vi "NanoDropInterp.vi"() -> ()   [LabVIEW 2022 SP3]
uses:
  <vilib>/gmath/NI_Gmath.lvlib
  <vilib>/Analysis/NI_AALPro.lvlib
  <vilib>/Analysis/NI_AALBase.lvlib
panel:
  in  "Threshol values":dbl[](array[numeric])=[20.0, 30.0]
  in  "delta":dbl
  in  "Cal":string="20\t-0.47978\n40\t-0.89772\n60\t-1.28062\n80\t-1.51509\n100\t-1.73927\n120\t-2.04589\n140\t-2.62307\n160\t-3.32393\n180\t-3.88565\n200\t-4.48344\n220\t-4.98332\n240\t-5.39044\n260\t-5.87486\n280\t-6.95707\n300\t-7.65792\n320\t-8.15265\n340\t-8.31756\n360\t-8.86382\n380\t-8.8329\n400\t-9.08026\n"
  out "Pressure threshold":dbl[][](array[numeric])
  out "Output to cut and paste":string
  out "Interp output":dbl[][](array[numeric])
  in  "shift":dbl
  in  "steps":i32
  in  "Paste tab data":string
  out "Input array":dbl[][](array[numeric])
  # "average and SD are last columns"
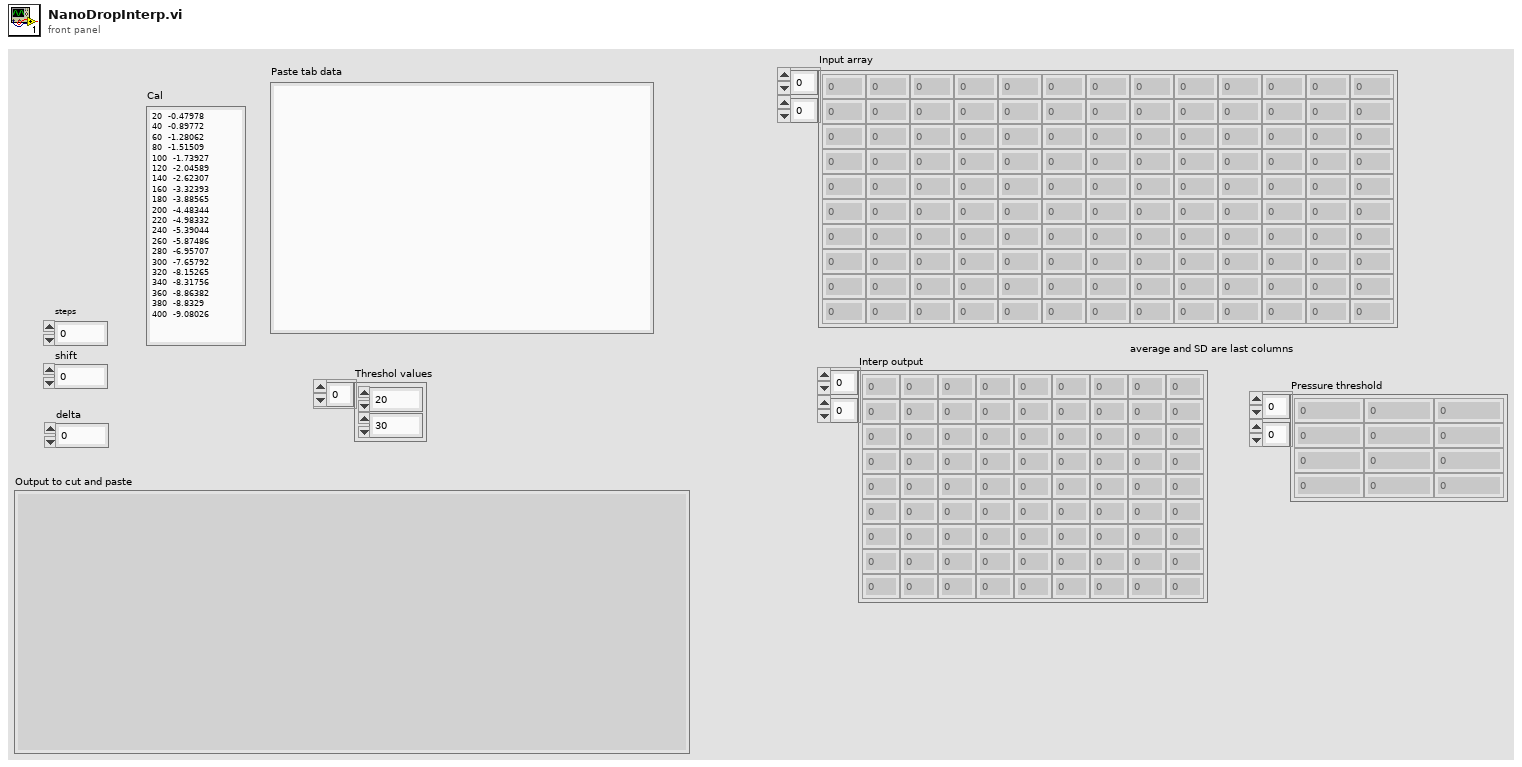
[diagram p1: front panel]
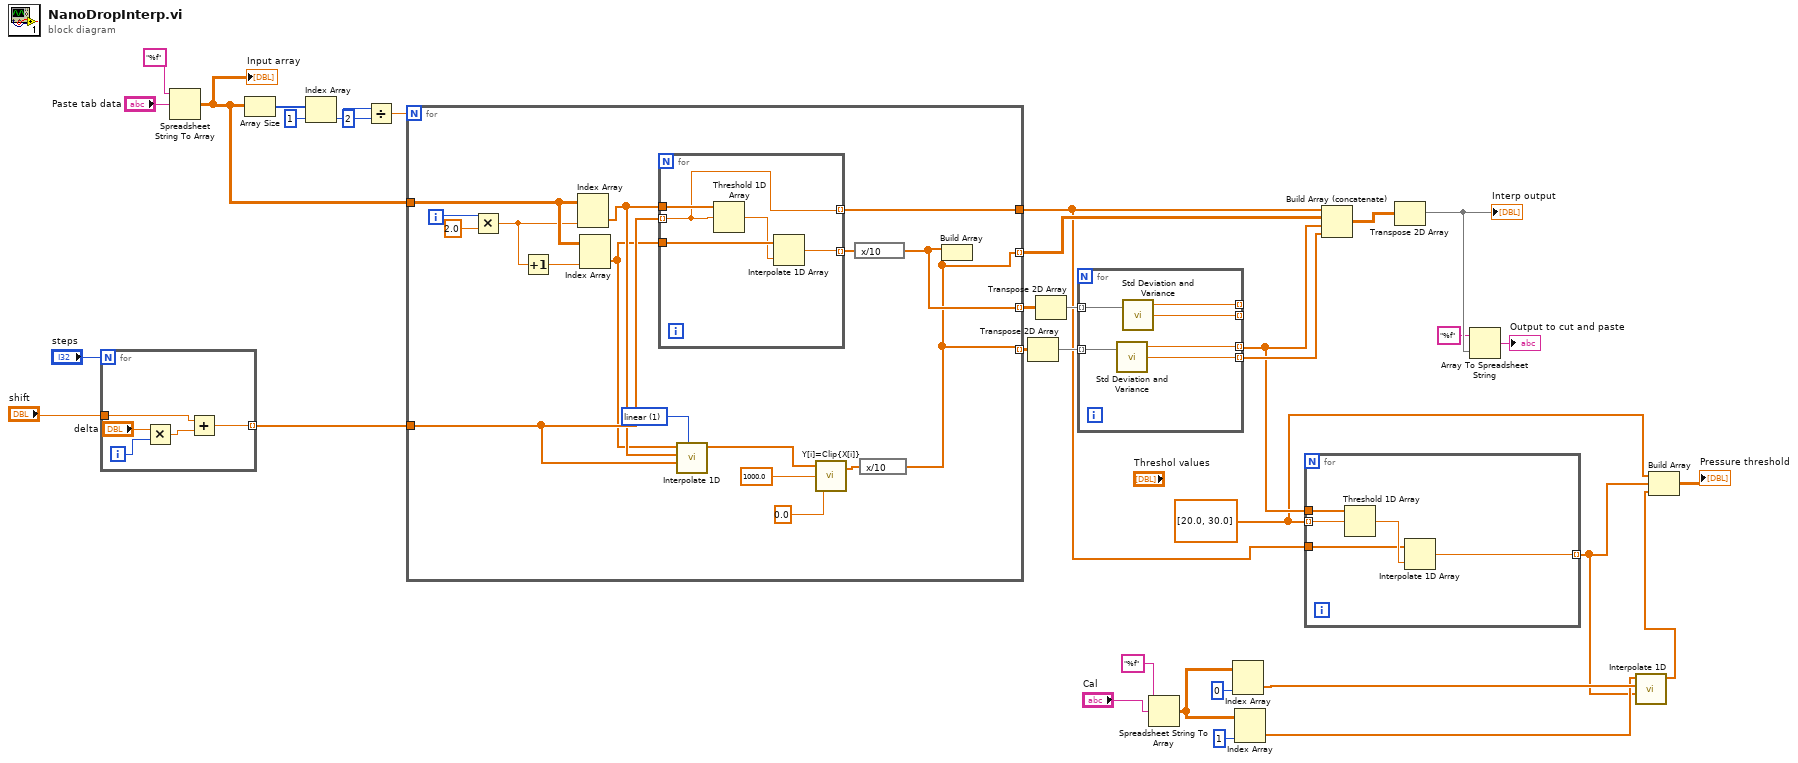
[diagram p0: block diagram]
diagram:
  w11 = dbl[] [20.0, 30.0]
  n1 = for {
    N: "steps" -> [_]
    tunnel: "shift" -> [w37]
    tunnel: [w36] -> w24 mode=indexing
    i -> [w39]
    n2 = Multiply(x="delta", y=w39) -> (x*y=w38:dbl)
    n3 = Add(x=w37, y=w38) -> (x+y=w36:dbl)
  }
  n4 = Spreadsheet String To Array(format string="%f", spreadsheet string="Paste tab data") -> (array=w27:dbl[][])  [unwired: 2 in]
  "Input array" <- w27
  n5 = Array Size(array=w27) -> (size(s)=w32:i32[])
  n6 = Index Array(array=w32, index=1) -> (element=w30:i32)
  n7 = Divide(x=w30, y=2) -> (x/y=w28:dbl)
  n8 = for {
    N: w28 -> [_]
    tunnel: w27 -> [w54]
    tunnel: w24 -> [w51]
    tunnel: [w40] -> w21 mode=indexing
    tunnel: [w40] -> w22 mode=indexing
    tunnel: [w42] -> w23 mode=indexing
    tunnel: [w44] -> w12
    i -> [w55]
    w41 = 1 items=["nearest", "linear", "spline", "cubic Hermite", "Lagrange"] ("method")
    n9 = Multiply(x=w55, y=2.0) -> (x*y=w53:dbl)
    n10 = Increment(x=w53) -> (x+1=w52:dbl)
    n11 = Index Array(array=w54, index (col)=w53) -> (element=w50:dbl[])  [unwired: 1 in]
    n12 = Index Array(array=w54, index (col)=w52) -> (element=w49:dbl[])  [unwired: 1 in]
    n13 = for {
      tunnel: w50 -> [w61]
      tunnel: w51 -> [w58] mode=indexing
      tunnel: w49 -> [w60]
      tunnel: [w59] -> w43 mode=indexing
      tunnel: [w58] -> w44 mode=indexing
      n14 = Threshold 1D Array(2:w58, 3:w61) -> (0:w57:dbl)  [unwired: 1 in]
      n15 = Interpolate 1D Array(1:w57, 2:w60) -> (0:w59:dbl)
    }
    n16 = call <vilib>:"Interpolate 1D.vi"("method"=w41, "xi"=w51, "X"=w50, "Y"=w49) -> ("yi"=w48:dbl[])  [unwired: 5 in, 2 out]
    n17 = call <vilib>:"Y[i]=Clip{X[i]}.vi"("lower limit"=0.0, "upper limit"=1000.0, "Input Array"=w48) -> ("Clipped Array"=w45:dbl[])  [unwired: 1 out]
    n18 = expression code="x/10"(w43) -> (w42:dbl[])
    n19 = expression code="x/10"(w45) -> (w40:dbl[])
    n20 = Build Array(w42, w40) -> ()  [unwired: 1 out]
  }
  n21 = Transpose 2D Array(2D array=w22) -> (transposed array=w18:dbl[][])
  n22 = Transpose 2D Array(2D array=w23) -> (transposed array=w19:dbl[][])
  n23 = for {
    tunnel: w19 -> [w67] mode=indexing
    tunnel: w18 -> [w66] mode=indexing
    tunnel: [w65] -> _ mode=indexing
    tunnel: [w64] -> w13 mode=indexing
    tunnel: [w63] -> _ mode=indexing
    tunnel: [w62] -> w16 mode=indexing
    n24 = call <vilib>:"Std Deviation and Variance.vi"("X"=w66) -> ("mean"=w64:dbl, "standard deviation"=w62:dbl)  [unwired: 1 in, 1 out]
    n25 = call <vilib>:"Std Deviation and Variance.vi"("X"=w67) -> ("mean"=w65:dbl, "standard deviation"=w63:dbl)  [unwired: 1 in, 1 out]
  }
  n26 = Spreadsheet String To Array(format string="%f", spreadsheet string="Cal") -> (array=w7:dbl[][])  [unwired: 2 in]
  n27 = Index Array(array=w7, index (col)=0 ("disabled index (col)")) -> (element=w6:dbl[])  [unwired: 1 in]
  n28 = Index Array(array=w7, index (col)=1 ("disabled index (col)")) -> (element=w5:dbl[])  [unwired: 1 in]
  n29 = for {
    tunnel: w13 -> [w71]
    tunnel: w11 -> [w70] mode=indexing
    tunnel: w12 -> [w69]
    tunnel: [w68] -> w4 mode=indexing
    n30 = Threshold 1D Array(2:w70, 3:w71) -> (0:w72:dbl)  [unwired: 1 in]
    n31 = Interpolate 1D Array(1:w72, 2:w69) -> (0:w68:dbl)
  }
  n32 = Build Array (concatenate)(w12, w21, w13, w16) -> (w20:dbl[][])
  n33 = Transpose 2D Array(2D array=w20) -> (transposed array=w17:dbl[][])
  "Interp output" <- w17
  n34 = Array To Spreadsheet String(array=w17, 3:"%f" ("format string")) -> (spreadsheet string=→"Output to cut and paste":string)  [unwired: 1 in]
  n35 = call <vilib>:"Interpolate 1D.vi"("xi"=w4, "X"=w6, "Y"=w5) -> ("yi"=w1:dbl[])  [unwired: 6 in, 2 out]
  n36 = Build Array(w11, w4, w1) -> (→"Pressure threshold":dbl[][])
